vi "Camera Manager.vi"   [LabVIEW 2011]
uses:
  Camera Data State.ctl
types:
  T1 = typedef "Camera Data State.ctl" = enum16{"Camera Conn Error (No Data)", "Dashboard Conn Error (Local Data)", "Dashboard Data"}
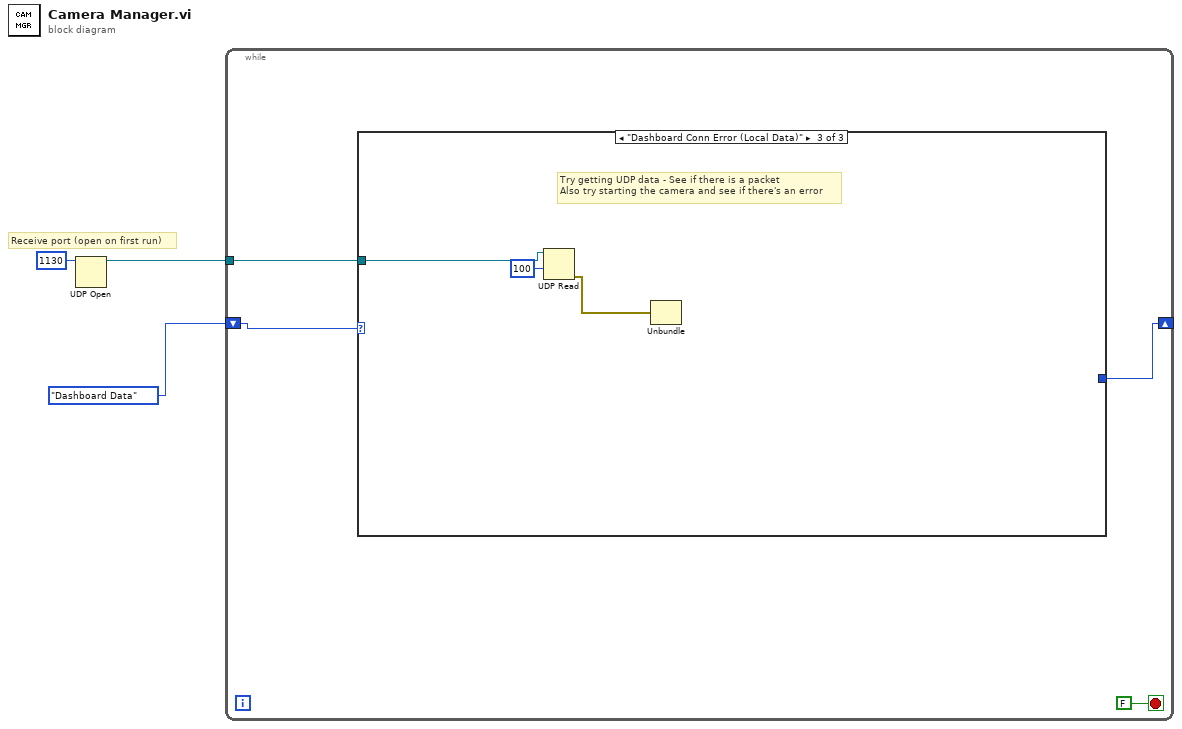
[diagram p0: block diagram]
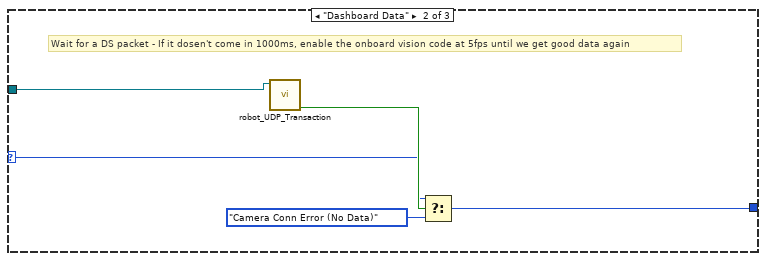
[diagram p3: hidden frame]
diagram:
  # "Receive port (open on first run)"
  n1 = UDP Open(11:u16 1130 ("port")) -> (port=w2:refnum<k16>)  [unwired: 4 in, 2 out]
  n2 = while {
    tunnel: w2 -> [w6]
    shift-right: [w4] -> _
    shift-left: Camera_Data_State."Dashboard Data" ("Camera Data State") -> [w5]
    stop <- FALSE stop-if-true
    n3 = case shown="\"Dashboard Conn Error (Local Data)\"" w5 {
      selector: w5 -> [_ w10 _]
      tunnel: w6 -> [_ w12 w15]
      tunnel: [_ w9 _] -> w4
      frame "Camera Conn Error (No Data)", Default {
      }
      frame "Dashboard Data" {
        # "Wait for a DS packet - If it dosen't come in 1000ms, enable the onboard vision code at 5fps until we get good data again"
        n4 = call "robot_UDP_Transaction.vi"("connection ID"=w12) -> ("status"=w11:bool)  [unwired: 9 in, 1 out]
        n5 = Select(t=w10, s=w11, f=Camera_Data_State."Camera Conn Error (No Data)") -> (s? t:f=w9:T1)
      }
      frame "Dashboard Conn Error (Local Data)" {
        # "Try getting UDP data - See if there is a packet\nAlso try starting the camera and see if there's an error"
        n6 = UDP Read(connection ID=w15, timeout ms (25000)=100) -> (error out=w13:errorcluster)  [unwired: 2 in, 4 out]
        n7 = Unbundle(w13) -> ()  [unwired: 3 out]
      }
    }
  }
